vi "SetTilecodeString.vi"(8 "error in (no error)":errorcluster, 10 "TileCode":string, 11 "PongSwitch in":refnum<class "SnakeSwitch.lvclass">) -> (0 "error out":errorcluster, 3 "PongSwitch out":refnum<class "SnakeSwitch.lvclass">)   [LabVIEW 2019, in "RT_Game.lvlib" / "SnakeSwitch.lvclass"]
uses:
  SnakeSwitch.lvclass
  SnakeSwitch.lvclass/SnakeSwitch.ctl
  Game/Game.lvclass
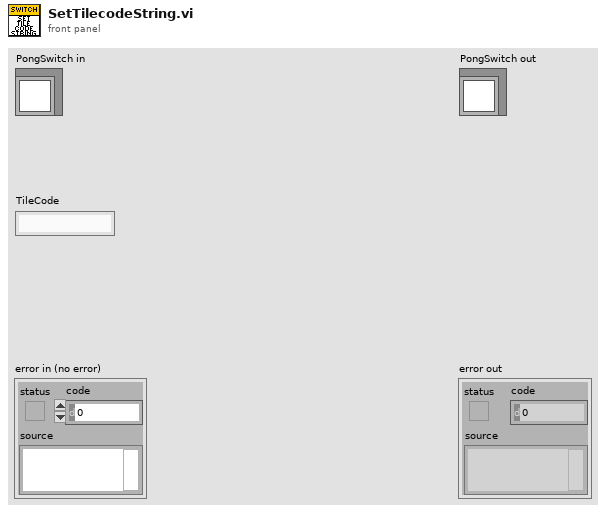
[diagram p1: front panel]
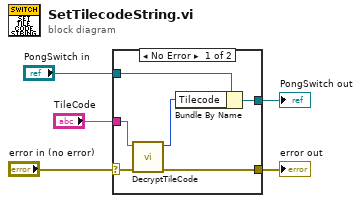
[diagram p0: block diagram]
diagram:
  n1 = case shown="No Error" "error in (no error)" {
    selector: "error in (no error)" -> [w11 w13]
    tunnel: [w9 w13] -> w4
    tunnel: [w7 w12] -> w2
    tunnel: "PongSwitch in" -> [w10 w12]
    tunnel: "TileCode" -> [w8 _]
    frame No Error {
      n2 = call "DecryptTileCode.vi"("error in (no error)"=w11, "TileCode"=w8) -> ("error out"=w9:errorcluster, "TileNumber"=w6:u16)  [unwired: 7 in, 1 out]
      n3 = Bundle By Name(cluster=w10, "Tilecode"=w6) -> (w7:refnum<class "SnakeSwitch.lvclass">)
    }
    frame Error {
    }
  }
  "error out" <- w4
  "PongSwitch out" <- w2
